vi "Maui.Config.ReadFramework.vi"(8 "error in (no error)":errorcluster, 10 "INI Fomatted Cluster Type":variant, 11 "Maui.Config in":refnum<class "Maui.Config.lvclass">) -> (0 "error out":errorcluster, 2 "INI Fomatted Cluster":variant, 3 "Maui.Config out":refnum<class "Maui.Config.lvclass">)   [LabVIEW 2019, in "Maui.Config.lvclass"]
uses:
  Maui.Config.lvclass
  <vilib>/Utility/config.llb/NI_LVConfig.lvlib
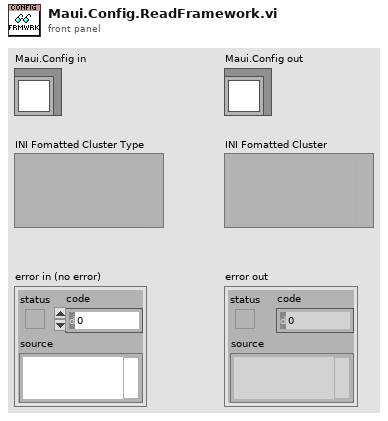
[diagram p1: front panel]
types:
  T1 = typedef "NI_LVConfig.lvlib/Config Data RefNum.ctl" = refnum<k1>
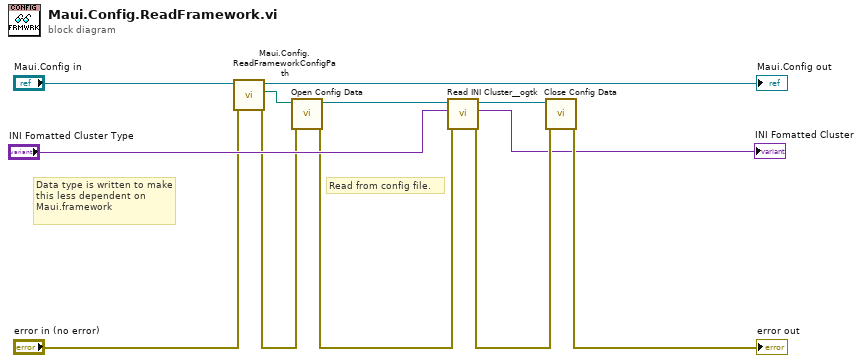
[diagram p0: block diagram]
diagram:
  # "Read from config file."
  # "Data type is written to make this less dependent on Maui.framework"
  n1 = call "Maui.Config.ReadFrameworkConfigPath.vi"("error in (no error)"="error in (no error)", "Maui.Config in"="Maui.Config in") -> ("error out"=w3:errorcluster, "Framework Configuration"=w2:path, "Maui.Config out"=→"Maui.Config out":refnum<class "Maui.Config.lvclass">)  [unwired: 7 in]
  n2 = call <vilib>:"Open Config Data.vi"("error in (no error)"=w3, "configuration file path"=w2) -> ("error out"=w8:errorcluster, "refnum"=w10:T1)  [unwired: 7 in, 1 out]
  n3 = call <userlib>:"Read INI Cluster__ogtk.vi"("error in (no error)"=w8, "INI Fomatted Cluster Type"="INI Fomatted Cluster Type", "refnum"=w10) -> ("error out"=w6:errorcluster, "INI Fomatted Cluster"=→"INI Fomatted Cluster":variant, "dup refnum"=w7:T1)  [unwired: 4 in, 2 out]
  n4 = call <vilib>:"Close Config Data.vi"("error in (no error)"=w6, "refnum"=w7) -> ("error out"=→"error out":errorcluster)  [unwired: 8 in, 1 out]
